vi "Measure_Voltage.vi"(6 "Resolution in Digits":T1(ring), 8 "error in (no error)":errorcluster, 9 "Range":dbl=1.2, 10 "Level":dbl, 11 "KeysightDmm in":refnum<class "KeysightDmm.lvclass"> caption="KeysightDMM in") -> (0 "error out":errorcluster, 1 "Out of Range":bool, 2 "DC_Voltage":dbl, 3 "KeysightDmm out":refnum<class "KeysightDmm.lvclass">)   [LabVIEW 2021, in "KeysightDmm.lvclass"]
uses:
  KeysightDmm.lvclass
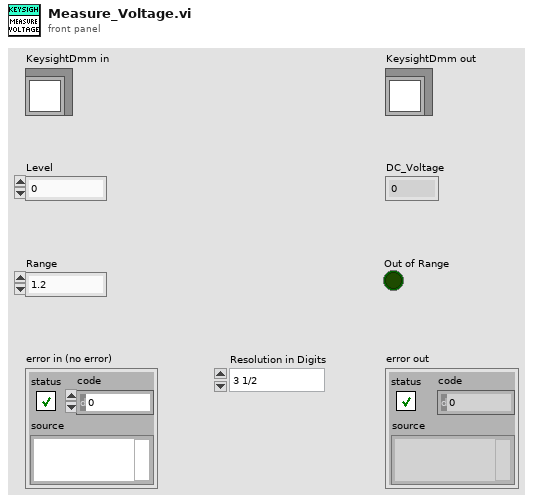
[diagram p1: front panel]
types:
  T1 = enum32{"3 1/2", "4 1/2", "5 1/2", "6 1/2", "7 1/2"}
  T2 = enum32{"DC Volts", "AC Volts", "DC Current", "AC Current", "2-wire Resistance", "4-wire Resistance", "Diode", "Frequency", "Period", "AC Volts DC Coupled", "Capacitance", "Inductance", "Temperature"}
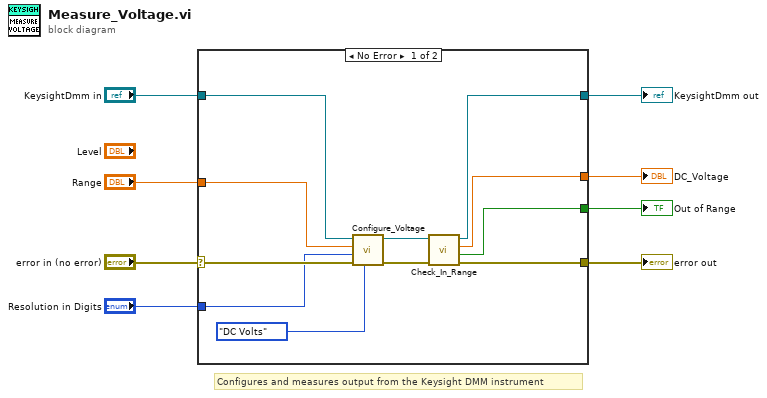
[diagram p0: block diagram]
diagram:
  # "Configures and measures output from the Keysight DMM instrument"
  n1 = case shown="No Error" "error in (no error)" {
    selector: "error in (no error)" -> [w19 w20]
    tunnel: "KeysightDmm in" -> [w13 w21]
    tunnel: [w10 w21] -> w7
    tunnel: [w16 w20] -> w5
    tunnel: "Resolution in Digits" -> [w18 _]
    tunnel: "Range" -> [w17 _]
    tunnel: [w15 _] -> w2
    tunnel: [w14 _] -> w1
    frame No Error {
      n2 = call "Configure_Voltage.vi"("Measurement Type"=T2."DC Volts", "error in (no error)"=w19, "Resolution in Digits"=w18, "Range"=w17, "KeysightDmm in"=w13) -> ("error out"=w12:errorcluster, "KeysightDmm out"=w11:refnum<class "KeysightDmm.lvclass">)  [unwired: 5 in]
      n3 = call "Check_In_Range.vi"("error in (no error)"=w12, "KeysightDmm in"=w11) -> ("error out"=w16:errorcluster, "Out_Of_Range"=w14:bool, "Measured_Value"=w15:dbl, "KeysightDmm out"=w10:refnum<class "KeysightDmm.lvclass">)  [unwired: 6 in]
    }
    frame Error {
    }
  }
  "error out" <- w5
  "KeysightDmm out" <- w7
  "DC_Voltage" <- w2
  "Out of Range" <- w1
